vi "ExampleGreyscaleImageData.vi"(1 "Image Size":T1={"Width"=256, "Height"=128}) -> (0 "GreyscaleImage":u8[][](array[numeric]))   [LabVIEW 2020, in "g_ar_toolkit.test.lvlib" / "Image.lvclass"]
uses:
  Image.lvclass
  g_ar_toolkit.image/Image Size (Fixed).ctl
  g_ar_toolkit.image/g_ar_toolkit.image.lvlib
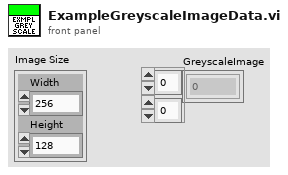
[diagram p1: front panel]
types:
  T1 = typedef "g_ar_toolkit.image.lvlib/Image Size (Fixed).ctl" = cluster{"Width":u16, "Height":u16}
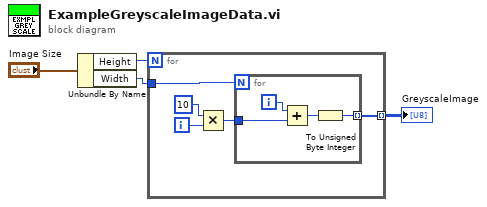
[diagram p0: block diagram]
diagram:
  n1 = Unbundle By Name("Image Size") -> ("Height"=w3:u16, "Width"=w2:u16)
  n2 = for {
    N: w3 -> [_]
    tunnel: w2 -> [w9]
    tunnel: [w5] -> w1 mode=indexing
    i -> [w8]
    n3 = Multiply(x=10, y=w8) -> (x*y=w6:i32)
    n4 = for {
      N: w9 -> [_]
      tunnel: w6 -> [w13]
      tunnel: [w10] -> w5 mode=indexing
      i -> [w12]
      n5 = Add(x=w12, y=w13) -> (x+y=w11:i32)
      n6 = To Unsigned Byte Integer(number=w11) -> (unsigned 8bit integer=w10:u8)
    }
  }
  "GreyscaleImage" <- w1
